vi "FTW-Benchmark-JSON.vi"() -> ()   [LabVIEW 2013]
uses:
  src/core/json/FTW-JSON-UpdateMode.ctl
  src/core/reflection/FTW-Reflection-Type.vi
  src/core/json/lib/FTW-JSON-Core-LibraryFilepath.vi
  src/core/json/lib/FTW-JSON-Core-GetFlattenedValue.vi
  src/core/json/lib/FTW-JSON-Core-LibraryError.vi
  src/core/json/FTW-JSON-Deserialize/FTW-JSON-Deserialize.xnode
  src/core/json/FTW-JSON.lvclass
panel:
  out "Results":T1(array[cluster]) {"Elapsed Time" format="%.6fsec"}
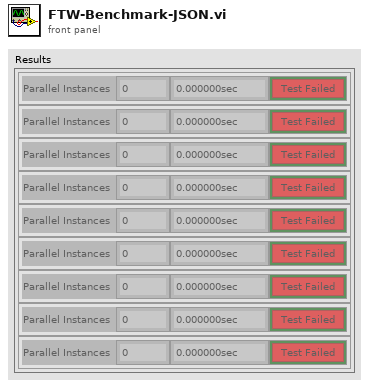
[diagram p1: front panel]
types:
  T1 = cluster{"Parallel Instances":i32, "Elapsed Time":dbl, bool}[]
  T2 = cluster{"LoggerDirectory":path, "Value":dbl, "LoggerAddress":string, "BooleanFalse":bool}
  T3 = typedef "FTW-JSON.lvclass/FTW-JSON-UpdateMode.ctl" = enum16{"Upsert", "Update Only", "Insert Only"}
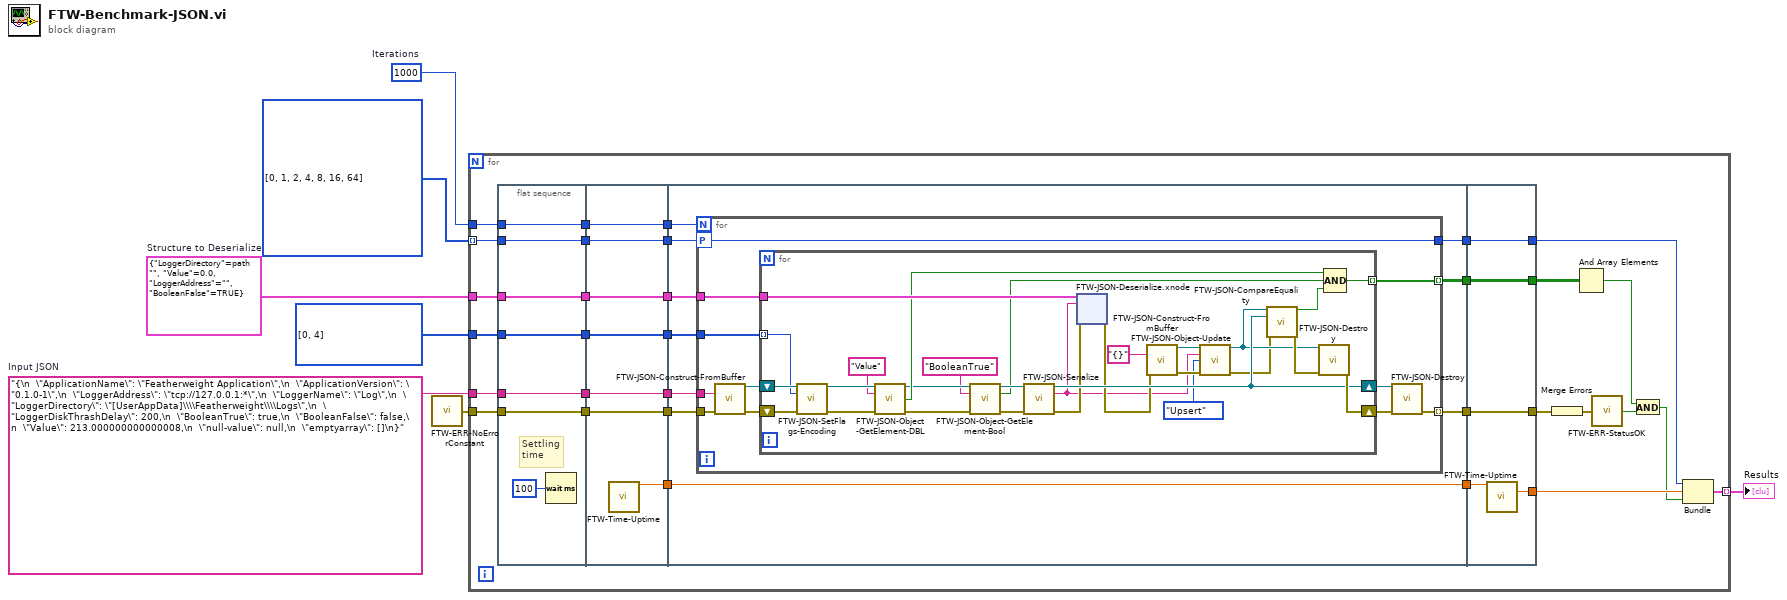
[diagram p0: block diagram]
diagram:
  w1 = T2 {"LoggerDirectory"=path "", "Value"=0.0, "LoggerAddress"="", "BooleanFalse"=TRUE}  # Structure to Deserialize
  w6 = "{\n  \"ApplicationName\": \"Featherweight Application\",\n  \"ApplicationVersion\": \"0.1.0-1\",\n  \"LoggerAddress\": \"tcp://127.0.0.1:*\",\n  \"LoggerName\": \"Log\",\n  \"LoggerDirectory\": \"[UserAppData]\\\\Featherweight\\\\Logs\",\n  \"LoggerDiskThrashDelay\": 200,\n  \"BooleanTrue\": true,\n  \"BooleanFalse\": false,\n  \"Value\": 213.000000000000008,\n  \"null-value\": null,\n  \"emptyarray\": []\n}"  # Input JSON
  w7 = 1000  # Iterations
  n1 = call "FTW-ERR-NoErrorConstant.vi"() -> ("no error"=w5:errorcluster)
  n2 = for {
    tunnel: w7 -> [w31]
    tunnel: w6 -> [w30]
    tunnel: w5 -> [w29]
    tunnel: i32[] [0, 4] -> [w28]
    tunnel: i32[] [0, 1, 2, 4, 8, 16, 64] -> [w24] mode=indexing
    tunnel: [w18] -> w2 mode=indexing
    tunnel: w1 -> [w10]
    n3 = flat-sequence {
      tunnel: w24 -> [w42]
      tunnel: w28 -> [w43]
      tunnel: w29 -> [w44]
      tunnel: w30 -> [w45]
      tunnel: w31 -> [w46]
      tunnel: [w46] -> w17
      tunnel: [w45] -> w16
      tunnel: [w44] -> w15
      tunnel: [w43] -> w14
      tunnel: [w42] -> w13
      tunnel: w10 -> [w40]
      tunnel: [w40] -> w9
      tunnel: [w53] -> w39
      tunnel: [w52] -> w38
      tunnel: [w51] -> w37
      tunnel: [w50] -> w36
      tunnel: [w49] -> w35
      tunnel: [w48] -> w27
      tunnel: w17 -> [w53]
      tunnel: w16 -> [w52]
      tunnel: w15 -> [w51]
      tunnel: w14 -> [w50]
      tunnel: w13 -> [w48]
      tunnel: w9 -> [w47]
      tunnel: [w47] -> w8
      tunnel: w39 -> [w63]
      tunnel: w38 -> [w55]
      tunnel: w37 -> [w61]
      tunnel: w36 -> [w59]
      tunnel: [w62] -> w34
      tunnel: [w60] -> w33
      tunnel: [w58] -> w32
      tunnel: w35 -> [w58]
      tunnel: w27 -> [w57]
      tunnel: [w56] -> w11
      tunnel: w8 -> [w54]
      tunnel: [w140] -> w23
      tunnel: [w141] -> w25
      tunnel: w34 -> [w141]
      tunnel: w33 -> [w140]
      tunnel: w32 -> [w139]
      tunnel: [w138] -> w26
      tunnel: [w137] -> w12
      tunnel: w11 -> [w137]
      frame #0 {
        # "Settling\ntime"
        n4 = Wait (ms)(milliseconds to wait=u32 100) -> ()  [unwired: 1 out]
      }
      frame #1 {
        n5 = call "FTW-Time-Uptime.vi"() -> ("Current Uptime"=w49:dbl)  [unwired: 13 in, 2 out]
      }
      frame #2 {
        n6 = for {
          N: w63 -> [_]
          tunnel: w55 -> [w72]
          tunnel: [w66] -> w60 mode=indexing
          tunnel: w59 -> [w67]
          workers-P: w57 -> [w65]
          tunnel: w61 -> [w74]
          tunnel: [w73] -> w62 mode=indexing
          tunnel: [w65] -> w56
          tunnel: w54 -> [w64]
          n7 = call "FTW-JSON-Construct-FromBuffer.vi"("JSON String (UTF-8)"=w72, "error in"=w74) -> ("JSON Object"=w68:refnum<class "FTW-JSON.lvclass">, "error out"=w69:errorcluster)  [unwired: 12 in]
          n8 = for {
            tunnel: w67 -> [w98] mode=indexing
            shift-right: [w97] -> w70
            shift-left: w68 -> [w99]
            shift-right: [w102] -> w71
            shift-left: w69 -> [w100]
            tunnel: [w90] -> w66 mode=indexing
            tunnel: w64 -> [w94]
            n9 = call "FTW-JSON-SetFlags-Encoding.vi"("JSON Object"=w99, "Indent Spaces"=w98, "error in"=w100) -> ("JSON Object out"=w93:refnum<class "FTW-JSON.lvclass">, "error out"=w92:errorcluster)  [unwired: 11 in]
            n10 = call "FTW-JSON-Object-GetElement-DBL.vi"("JSON Object"=w93, "Key"="Value", "error in"=w92) -> ("JSON Object out"=w85:refnum<class "FTW-JSON.lvclass">, "Found?"=w91:bool, "error out"=w84:errorcluster)  [unwired: 9 in, 1 out]
            n11 = call "FTW-JSON-Object-GetElement-Bool.vi"("JSON Object"=w85, "Key"="BooleanTrue", "error in"=w84) -> ("JSON Object out"=w89:refnum<class "FTW-JSON.lvclass">, "Value"=w87:bool, "error out"=w88:errorcluster)  [unwired: 9 in, 1 out]
            n12 = call "FTW-JSON-Serialize.vi"("JSON Object"=w89, "error in"=w88) -> ("JSON Object out"=w97:refnum<class "FTW-JSON.lvclass">, "JSON String (UTF-8)"=w76:string, "error out"=w96:errorcluster)  [unwired: 11 in]
            n13 = xnode "FTW-JSON-Deserialize.xnode"("Type and Defaults"=w94, "JSON String"=w76, "error in"=w96) -> ("error out"=w95:errorcluster)  [unwired: 1 out]
            n14 = call "FTW-JSON-Construct-FromBuffer.vi"("JSON String (UTF-8)"="{}", "error in"=w95) -> ("JSON Object"=w80:refnum<class "FTW-JSON.lvclass">, "error out"=w78:errorcluster)  [unwired: 12 in]
            n15 = call "FTW-JSON-Object-Update.vi"("JSON Object"=w80, "JSON Object to Merge"=w76, "Update Mode"=FTW-JSON-UpdateMode."Upsert", "error in"=w78) -> ("JSON Object out"=w79:refnum<class "FTW-JSON.lvclass">, "error out"=w77:errorcluster)  [unwired: 10 in]
            n16 = call "FTW-JSON-CompareEquality.vi"("JSON Object"=w79, "JSON Object to Compare"=w97, "error in"=w77) -> ("Equal?"=w82:bool, "error out"=w101:errorcluster)  [unwired: 11 in]
            n17 = call "FTW-JSON-Destroy.vi"("JSON Object"=w79, "error in"=w101) -> ("error out"=w102:errorcluster)  [unwired: 13 in]
            n18 = Compound Arithmetic op=AND(w91, w87, w82) -> (w90:bool)
          }
          n19 = call "FTW-JSON-Destroy.vi"("JSON Object"=w70, "error in"=w71) -> ("error out"=w73:errorcluster)  [unwired: 13 in]
        }
      }
      frame #3 {
        n20 = call "FTW-Time-Uptime.vi"("Previous Uptime"=w139) -> ("Elapsed Time"=w138:dbl)  [unwired: 12 in, 2 out]
      }
    }
    n21 = Merge Errors(w25) -> (w22:errorcluster)
    n22 = And Array Elements(Boolean array=w23) -> (logical AND=w20:bool)
    n23 = call "FTW-ERR-StatusOK.vi"("error to check"=w22) -> ("Status OK?"=w21:bool)
    n24 = And(x=w20, y=w21) -> (x .and. y?=w19:bool)
    n25 = Bundle(w12, "Elapsed Time"=w26, w19) -> (w18:cluster{i32, "Elapsed Time":dbl, bool})  [unwired: 1 in]
  }
  "Results" <- w2
